vi "chord length.vi"(2 "theta":dbl, 3 "arc length":dbl) -> (1 "chord length":dbl)   [LabVIEW 2009]
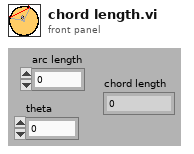
[diagram p1: front panel]
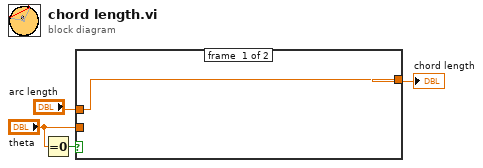
[diagram p0: block diagram]
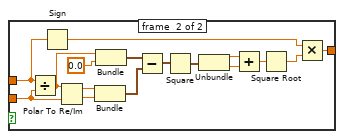
[diagram p2: hidden frame]
diagram:
  n1 = Equal To 0?(x="theta") -> (x = 0?=w1:bool)
  n2 = case shown="False" w1 {
    tunnel: "arc length" -> [w5 w9]
    tunnel: "theta" -> [_ w20]
    tunnel: [w5 w6] -> w3
    frame #0 {
    }
    frame #1 {
      n3 = Divide(x=w9, y=w20) -> (x/y=w12:dbl)
      n4 = Sign(1:w9) -> (0:w8:dbl)
      n5 = Polar To Re/Im(2:w20, 3:w12) -> (0:w18:dbl, 1:w19:dbl)
      n6 = Bundle(w19, w18) -> (w16:cluster{dbl, dbl})  [unwired: 1 in]
      n7 = Bundle(w12, "theta"=0.0) -> (w10:cluster{dbl, "theta":dbl})  [unwired: 1 in]
      n8 = Subtract(x=w10, y=w16) -> (x-y=w17:cluster{dbl, dbl})
      n9 = Square(x=w17) -> (x^2=w15:cluster{dbl, dbl})
      n10 = Unbundle(w15) -> (w14:dbl, w13:dbl)
      n11 = Add(x=w14, y=w13) -> (x+y=w21:dbl)
      n12 = Square Root(x=w21) -> (sqrt(x)=w7:dbl)
      n13 = Multiply(x=w8, y=w7) -> (x*y=w6:dbl)
    }
  }
  "chord length" <- w3
